vi "Get Platano Name.vi"(8 "error in (no error)":errorcluster, 11 "Platano in":refnum<class "Platano.lvclass">) -> (0 "error out":errorcluster, 2 "Varietal":string, 3 "Platano out":refnum<class "Platano.lvclass">)   [LabVIEW 2021, in "Bananas.lvlib" / "Platano.lvclass"]
uses:
  Platano.lvclass
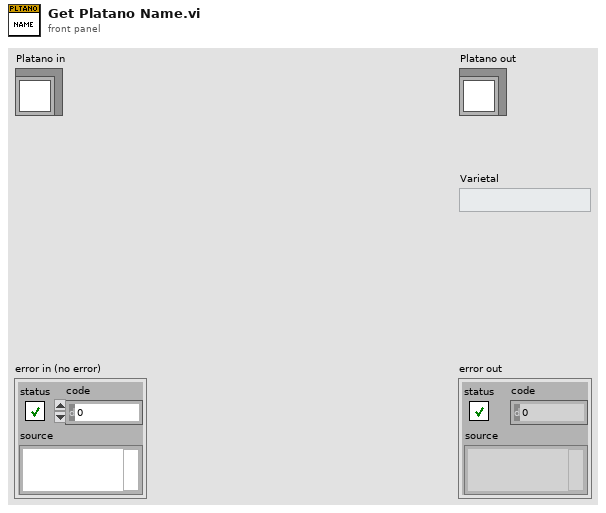
[diagram p1: front panel]
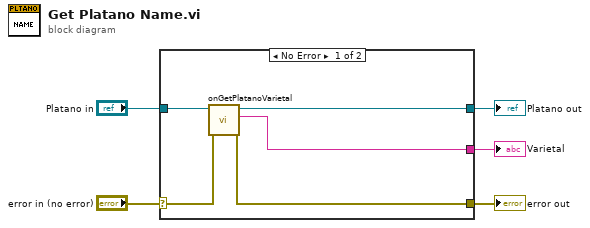
[diagram p0: block diagram]
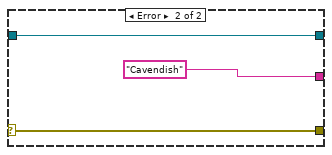
[diagram p2: hidden frame]
diagram:
  n1 = case shown="No Error" "error in (no error)" {
    selector: "error in (no error)" -> [w8 w13]
    tunnel: [w7 w13] -> w4
    tunnel: [w10 w12] -> w2
    tunnel: "Platano in" -> [w9 w12]
    tunnel: [w6 "Cavendish" ("Varietal")] -> w1
    frame No Error {
      n2 = call-dynamic "onGetPlatanoVarietal.vi"("error in (no error)"=w8, "Platano in"=w9) -> ("error out"=w7:errorcluster, "Varietal"=w6:string, "Platano out"=w10:refnum<class "Platano.lvclass">)  [unwired: 7 in]
    }
    frame Error {
    }
  }
  "error out" <- w4
  "Platano out" <- w2
  "Varietal" <- w1
